vi "Read Server RPC Methods.vi"(8 "error in (no error)":errorcluster, 11 "SignalGeneratorService in":refnum<class "MeasurementServiceBaseV2.lvclass">) -> (0 "error out":errorcluster, 2 "Server RPC Methods":T1, 3 "SignalGeneratorService out":refnum<class "MeasurementServiceBaseV2.lvclass">)   [LabVIEW 2020, in "MeasurementLink Measurement Service Base V2.lvlib" / "MeasurementServiceBaseV2.lvclass"]
uses:
  MeasurementServiceBaseV2.lvclass
  typeDefs/Server gRPC UEs.ctl
  <vilib>/gRPC/LabVIEW gRPC Library/Server API/typeDefs/gRPCId Cluster.ctl
  <vilib>/gRPC/LabVIEW gRPC Library/Shared/grpcId.ctl
  MeasurementServiceBaseV2.lvclass/MeasurementServiceBaseV2.ctl
  <vilib>/gRPC/LabVIEW gRPC Library/grpc-lvsupport-release.lvlib
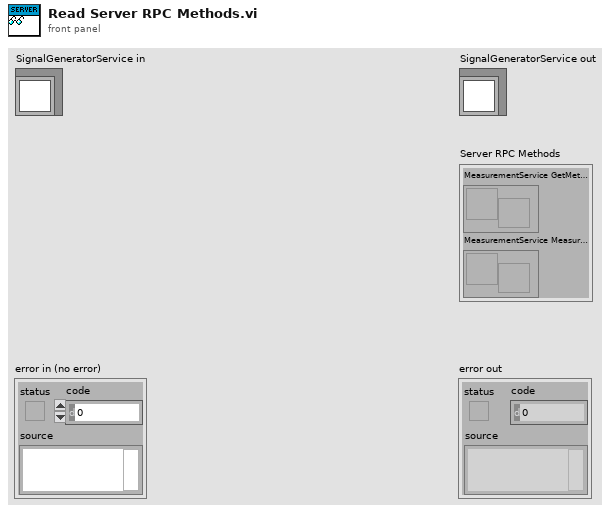
[diagram p1: front panel]
types:
  T1 = typedef "MeasurementLink Measurement Service Base V2.lvlib/MeasurementServiceBaseV2.lvclass/Server gRPC UEs.ctl" = cluster{"MeasurementService GetMetadata gRPC UE":refnum<user-event>, "MeasurementService Measure gRPC UE":refnum<user-event>}
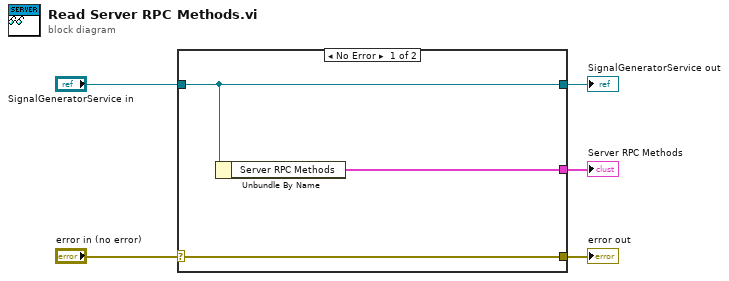
[diagram p0: block diagram]
diagram:
  n1 = case shown="No Error" "error in (no error)" {
    selector: "error in (no error)" -> [w8 w9]
    tunnel: [w8 w9] -> w4
    tunnel: [w7 w10] -> w2
    tunnel: "SignalGeneratorService in" -> [w7 w10]
    tunnel: [w6 _] -> w1
    frame No Error {
      n2 = Unbundle By Name(w7) -> ("Server RPC Methods"=w6:T1)
    }
    frame Error {
    }
  }
  "error out" <- w4
  "SignalGeneratorService out" <- w2
  "Server RPC Methods" <- w1
